vi "test_Read Command.vi"(8 "error in (no error)":errorcluster, 10 "t_ Host to Target":u64, 11 "Generator Data in":T1) -> (0 "error out":errorcluster, 2 "Monitor Enable?":bool, 3 "Generator Data out":T1)   [LabVIEW 2016]
uses:
  FPGA/Typedefs/Generator Data Cluster.ctl
  Host/Typedefs/IO Buffer Operation.ctl
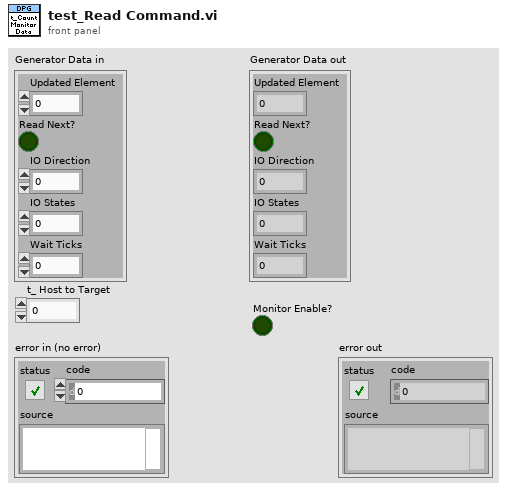
[diagram p1: front panel]
types:
  T1 = typedef "Generator Data Cluster.ctl" = cluster{"Updated Element":u64, "Read Next?":bool, "IO Direction":u32, "IO States":u32, "Wait Ticks":u32}
  T2 = typedef "IO Buffer Operation.ctl" = enum16{"Initialize", "Write IO Data_Rd", "Read IO Data_Rd", "Write IO Data_Wr", "Read IO Data_Wr", "Write  IO Data_Dir", "Read  IO Data_Dir", "Write Host to Target FIFO", "Read Host to Target FIFO", "Write Target to Host FIFO", "Read Target to Host FIFO", "Write Monitor Enable?", "Read Monitor Enable?", "Close"}
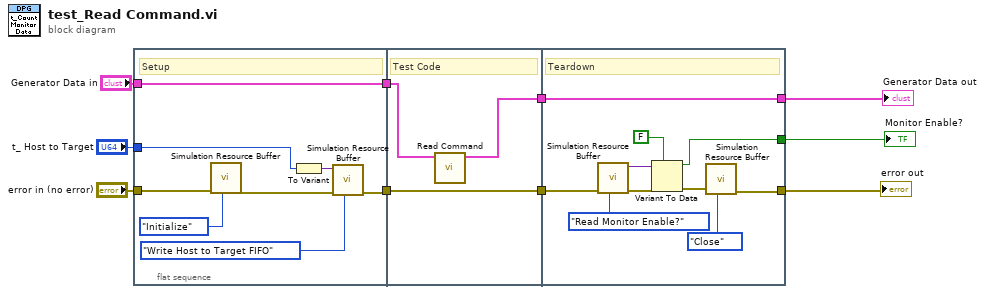
[diagram p0: block diagram]
diagram:
  n1 = flat-sequence {
    tunnel: "error in (no error)" -> [w14]
    tunnel: [w16] -> w8
    tunnel: "t_ Host to Target" -> [w15]
    tunnel: [w12] -> w4
    tunnel: "Generator Data in" -> [w12]
    tunnel: w8 -> [w21]
    tunnel: [w21] -> w6
    tunnel: [w20] -> w5
    tunnel: w4 -> [w19]
    tunnel: [w31] -> w10
    tunnel: w6 -> [w28]
    tunnel: [w29] -> w2
    tunnel: w5 -> [w29]
    tunnel: [w22] -> w1
    frame #0 {
      # "Setup"
      n2 = call "Simulation Resource Buffer.vi"("IO Buffer Operation"=IO_Buffer_Operation."Initialize", "error in (no error)"=w14) -> ("error out"=w11:errorcluster)  [unwired: 7 in, 2 out]
      n3 = To Variant(anything=w15) -> (Variant=w17:variant)
      n4 = call "Simulation Resource Buffer.vi"("IO Buffer Operation"=IO_Buffer_Operation."Write Host to Target FIFO", "error in (no error)"=w11, "Data in"=w17) -> ("error out"=w16:errorcluster)  [unwired: 6 in, 2 out]
    }
    frame #1 {
      # "Test Code"
      n5 = call "Read Command.vi"("Generator Data in"=w19) -> ("Generator Data out"=w20:T1)  [unwired: 10 in]
    }
    frame #2 {
      # "Teardown"
      n6 = call "Simulation Resource Buffer.vi"("IO Buffer Operation"=IO_Buffer_Operation."Read Monitor Enable?", "error in (no error)"=w28) -> ("error out"=w26:errorcluster, "Data out"=w25:variant)  [unwired: 7 in, 1 out]
      n7 = Variant To Data(error in=w26, type=FALSE, Variant=w25) -> (data=w22:bool, error out=w24:errorcluster)
      n8 = call "Simulation Resource Buffer.vi"("IO Buffer Operation"=IO_Buffer_Operation."Close", "error in (no error)"=w24) -> ("error out"=w31:errorcluster)  [unwired: 7 in, 2 out]
    }
  }
  "error out" <- w10
  "Generator Data out" <- w2
  "Monitor Enable?" <- w1
